vi "Configure Inrush Current Measurement.vi"(8 "error in (no error)":errorcluster, 9 "Inrush Current Interval (0 ms)":u32 max=10000, 10 "Inrush Current Start (0 ms)":u32 max=10000, 11 "VISA resource name":refnum<visa-resource-name>) -> (0 "error out":errorcluster, 3 "VISA resource name out":refnum<visa-resource-name>)   [LabVIEW 2015, in "BK Precision 983X Series.lvlib"]
doc: "Configures the inrush current measurement settings."
uses:
  <instrlib>/BK Precision 983X Series/BK Precision 983X Series.lvlib
panel:
  # "ms"
  # "ms"
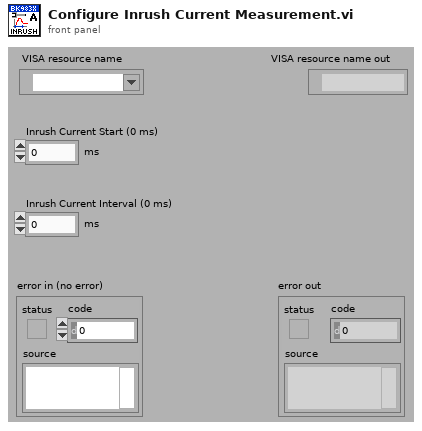
[diagram p1: front panel]
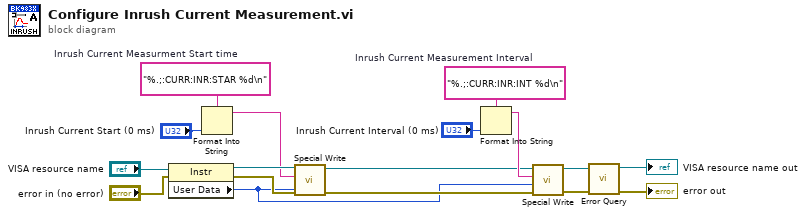
[diagram p0: block diagram]
diagram:
  w11 = "%.;:CURR:INR:INT %d\n"  # Inrush Current Measurement Interval
  w15 = "%.;:CURR:INR:STAR %d\n"  # Inrush Current Measurment Start time
  n1 = property class="Instr"(reference="VISA resource name", error in="error in (no error)") -> (reference out=w6:refnum<visa-resource-name>, error out=w5:errorcluster, "User Data"=w1:u32)
  n2 = Format Into String(format string=w15, "Inrush Current Start (0 ms)") -> (resulting string=w4:string)  [unwired: 2 in, 1 out]
  n3 = call <instrlib>:"Special Write.vi"("error in (no error)"=w5, "Delay (0 ms)"=w1, "Input String"=w4, "VISA resource name"=w6) -> ("error out"=w2:errorcluster, "VISA resource name out"=w3:refnum<visa-resource-name>)  [unwired: 6 in]
  n4 = Format Into String(format string=w11, "Inrush Current Interval (0 ms)") -> (resulting string=w9:string)  [unwired: 2 in, 1 out]
  n5 = call <instrlib>:"Special Write.vi"("error in (no error)"=w2, "Delay (0 ms)"=w1, "Input String"=w9, "VISA resource name"=w3) -> ("error out"=w7:errorcluster, "VISA resource name out"=w8:refnum<visa-resource-name>)  [unwired: 6 in]
  n6 = call <instrlib>:"Error Query.vi"("error in (no error)"=w7, "VISA resource name"=w8) -> ("error out"=→"error out":errorcluster, "VISA resource name out"=→"VISA resource name out":refnum<visa-resource-name>)  [unwired: 6 in, 2 out]
